vi "Signal Generator by Duration.vi"(0 "signal type":T1(ring), 2 "duration":dbl=1.0 format="%0.2f", 3 "reset phase":bool=TRUE, 5 "# of samples":i32=100, 7 "frequency":dbl=10.0 format="%0.2f", 9 "amplitude":dbl=1.0 format="%0.2f", 11 "dc offset":dbl format="%0.2f", 12 "phase in":dbl format="%0.2f", 13 "square wave duty cycle (%)":dbl=50.0 format="%0.2f") -> (4 "signal":dbl[](array[numeric]), 10 "sample rate":dbl=1.0 format="%0.2f", 14 "phase out":dbl format="%0.2e", 15 "error":i32)   [LabVIEW 2010, in "NI_AALPro.lvlib"]
doc: "Generates a <B>signal</B> with a shape given by the <B>signal type</B>."
uses:
  NI_AALPro.lvlib
  Ramp Pattern by Samples.vi
  NI_AALBase.lvlib
panel:
  # "Signal Generator by Duration"
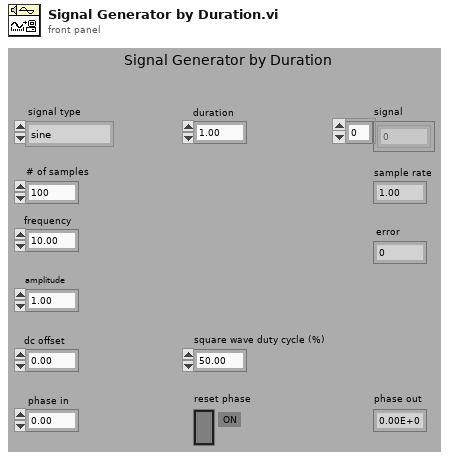
[diagram p1: front panel]
types:
  T1 = enum16{"sine", "cosine", "triangle", "square", "sawtooth", "increasing ramp", "decreasing ramp"}
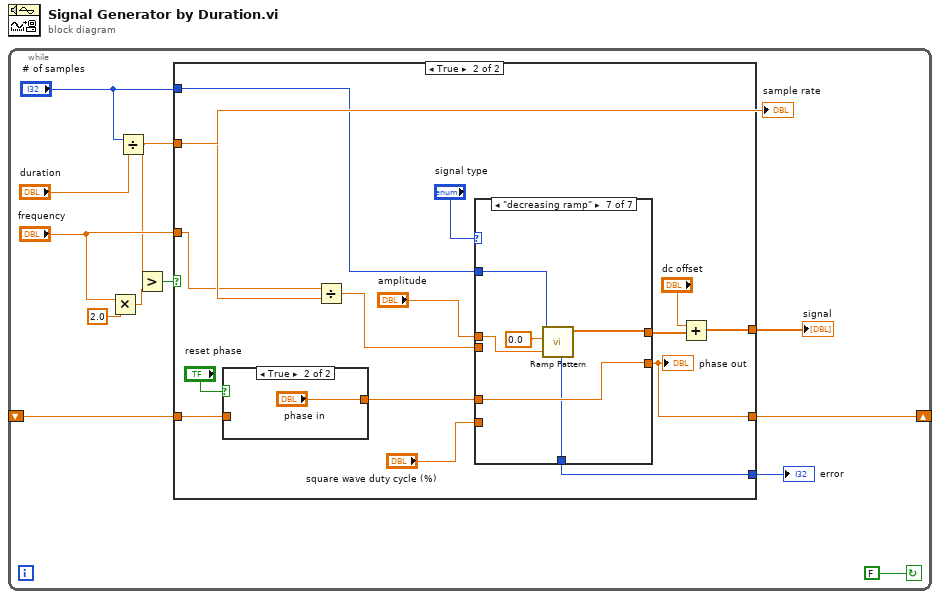
[diagram p0: block diagram]
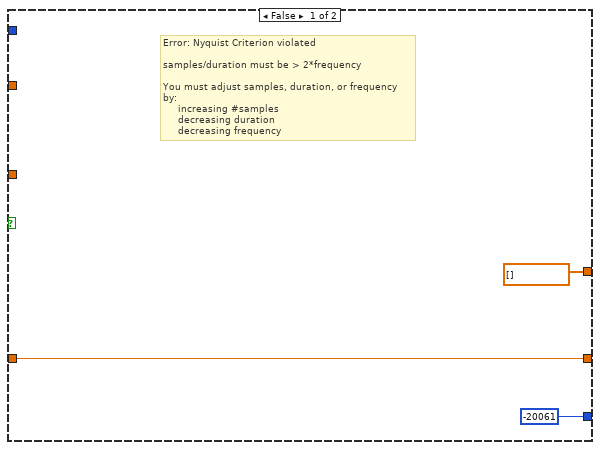
[diagram p2: hidden frame]
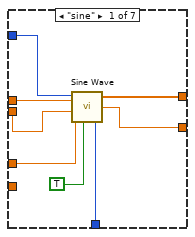
[diagram p4: hidden frame]
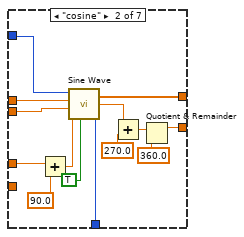
[diagram p5: hidden frame]
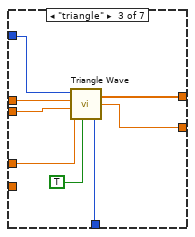
[diagram p6: hidden frame]
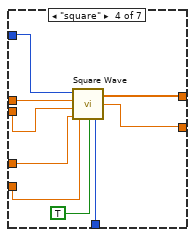
[diagram p7: hidden frame]
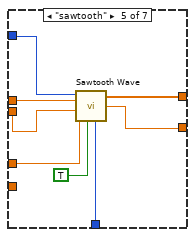
[diagram p8: hidden frame]
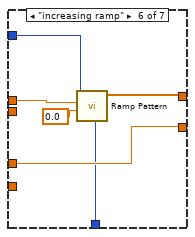
[diagram p9: hidden frame]
diagram:
  n1 = while {
    shift-left: _ -> [w12]
    shift-right: [w11] -> _
    stop <- FALSE continue-if-true
    n2 = Multiply(x="frequency", y=2.0) -> (x*y=w5:dbl)
    n3 = Divide(x="# of samples", y="duration") -> (x/y=w4:dbl)
    "sample rate" <- w4
    n4 = Greater?(x=w4, y=w5) -> (0:w3:bool)
    n5 = case shown="True" w3 {
      tunnel: w4 -> [_ w30]
      tunnel: "# of samples" -> [_ w29]
      tunnel: "frequency" -> [_ w27]
      tunnel: [-20061 ("error") w24] -> w10
      tunnel: [w13 w21] -> w11
      tunnel: w12 -> [w13 w17]
      tunnel: [dbl[] [] ("Signal") w16] -> w1
      frame False {
        # "Error: Nyquist Criterion violated\n\nsamples/duration must be > 2*frequency\n\nYou must adjust samples, duration, or frequency by:\n     increasing #samples\n     decreasing duration\n     decreasing frequency"
      }
      frame True {
        n6 = case shown="True" "reset phase" {
          tunnel: [w31 "phase in"] -> w23
          tunnel: w17 -> [w31 _]
          frame False {
          }
          frame True {
          }
        }
        n7 = Divide(x=w27, y=w30) -> (x/y=w28:dbl)
        n8 = case shown="\"decreasing ramp\"" "signal type" {
          tunnel: "amplitude" -> [w40 w54 w62 w71 w73 w84 w88]
          tunnel: w23 -> [w39 w47 w61 w70 w79 w81 w87]
          tunnel: [w38 w49 w56 w64 w74 w82 w90] -> w25
          tunnel: w29 -> [w37 w52 w59 w68 w78 w85 w91]
          tunnel: w28 -> [w36 w53 w60 w69 w76 _ _]
          tunnel: [w35 w42 w58 w67 w77 w81 w87] -> w21
          tunnel: "square wave duty cycle (%)" -> [_ _ _ w66 _ _ _]
          tunnel: [w33 w46 w55 w63 w72 w80 w86] -> w24
          frame "sine" {
            n9 = call "Sine Wave.vi"("samples"=w37, "amplitude"=w40, "frequency"=w36, "phase in"=w39, "reset phase"=TRUE) -> ("sine wave"=w38:dbl[], "phase out"=w35:dbl, "error"=w33:i32)
          }
          frame "cosine" {
            n10 = Add(x=w47, y=90.0) -> (x+y=w50:dbl)
            n11 = call "Sine Wave.vi"("samples"=w52, "amplitude"=w54, "frequency"=w53, "phase in"=w50, "reset phase"=TRUE) -> ("sine wave"=w49:dbl[], "phase out"=w44:dbl, "error"=w46:i32)
            n12 = Add(x=w44, y=270.0) -> (x+y=w41:dbl)
            n13 = Quotient & Remainder(x=w41, y=360.0) -> (x-y*floor(x/y)=w42:dbl)  [unwired: 1 out]
          }
          frame "triangle" {
            n14 = call "Triangle Wave.vi"("samples"=w59, "amplitude"=w62, "frequency"=w60, "phase in"=w61, "reset phase"=TRUE) -> ("triangle wave"=w56:dbl[], "phase out"=w58:dbl, "error"=w55:i32)
          }
          frame "square" {
            n15 = call "Square Wave.vi"("samples"=w68, "reset phase"=TRUE, "amplitude"=w71, "frequency"=w69, "duty cycle (%)"=w66, "phase in"=w70) -> ("square wave"=w64:dbl[], "phase out"=w67:dbl, "error"=w63:i32)
          }
          frame "sawtooth" {
            n16 = call "Sawtooth Wave.vi"("samples"=w78, "amplitude"=w73, "frequency"=w76, "phase in"=w79, "reset phase"=TRUE) -> ("sawtooth wave"=w74:dbl[], "phase out"=w77:dbl, "error"=w72:i32)
          }
          frame "increasing ramp" {
            n17 = call-poly "Ramp Pattern.vi"("start"=0.0, "end"=w84, "samples"=w85) -> ("error"=w80:i32, "Ramp Pattern"=w82:dbl[])  [unwired: 7 in]
          }
          frame "decreasing ramp" {
            n18 = call-poly "Ramp Pattern.vi"("start"=w88, "end"=0.0 ("start"), "samples"=w91) -> ("error"=w86:i32, "Ramp Pattern"=w90:dbl[])  [unwired: 7 in]
          }
        }
        "phase out" <- w21
        n19 = Add(x="dc offset", y=w25) -> (x+y=w16:dbl[])
      }
    }
    "error" <- w10
    "signal" <- w1
  }
